vi "Excute.vi"(8 "error in (no error)":errorcluster, 11 "Invoker in":refnum<class "Invoker.lvclass">) -> (0 "error out":errorcluster, 3 "Invoker out":refnum<class "Invoker.lvclass">)   [LabVIEW 2014, in "Invoker.lvclass"]
uses:
  Invoker.lvclass
  Invoker.lvclass/Invoker.ctl
  Command/Command.lvclass
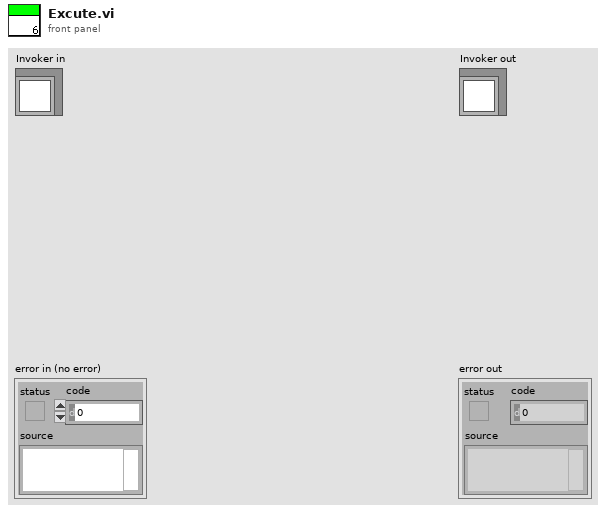
[diagram p1: front panel]
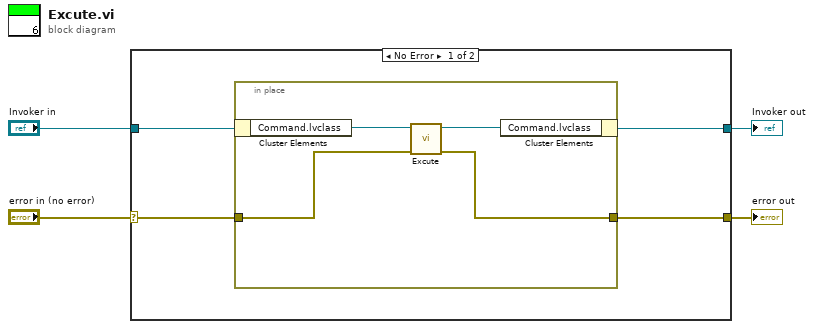
[diagram p0: block diagram]
diagram:
  n1 = case shown="No Error" "error in (no error)" {
    selector: "error in (no error)" -> [w6 w14]
    tunnel: [w5 w14] -> w3
    tunnel: [w7 w13] -> w1
    tunnel: "Invoker in" -> [w8 w13]
    frame No Error {
      n2 = in-place {
        in-place-border: w6 -> [w10]
        in-place-border: [w9] -> w5
        n3 = in-place-cluster #1(w8) -> ("Command.lvclass"=w12:refnum<class "Command.lvclass">)
        n4 = call-dynamic "Excute.vi"("error in (no error)"=w10, "Command in"=w12) -> ("error out"=w9:errorcluster, "Command out"=w11:refnum<class "Command.lvclass">)  [unwired: 8 in]
        n5 = in-place-cluster #1("Command.lvclass"=w11) -> (w7:refnum<class "Invoker.lvclass">)
      }
    }
    frame Error {
    }
  }
  "error out" <- w3
  "Invoker out" <- w1
